vi "Read Module Name.vi"(8 "error in (no error)":errorcluster, 11 "ADAS_IO_Template_MDO in":refnum<class "ADAS_IO_Template_MDO.lvclass">) -> (0 "error out":errorcluster, 2 "Module Name":string, 3 "ADAS_IO_Template_MDO out":refnum<class "ADAS_IO_Template_MDO.lvclass">)   [LabVIEW 2020, in "ADAS_IO_Template_MDO.lvclass"]
uses:
  ADAS_IO_Template_MDO.lvclass
  ADAS_IO_Template_MDO.lvclass/ADAS_IO_Template_MDO.ctl
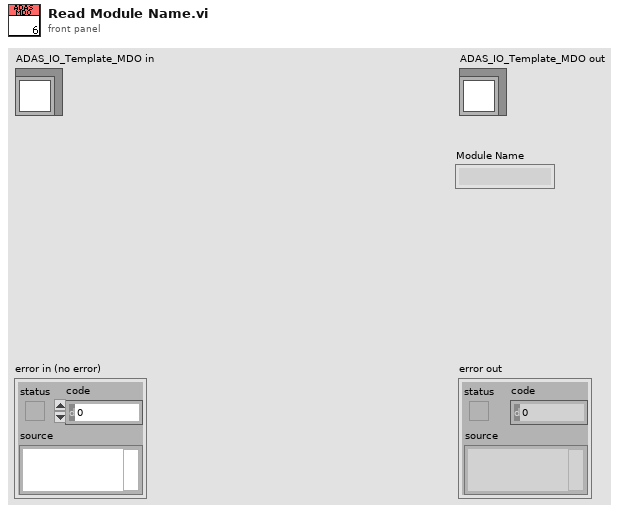
[diagram p1: front panel]
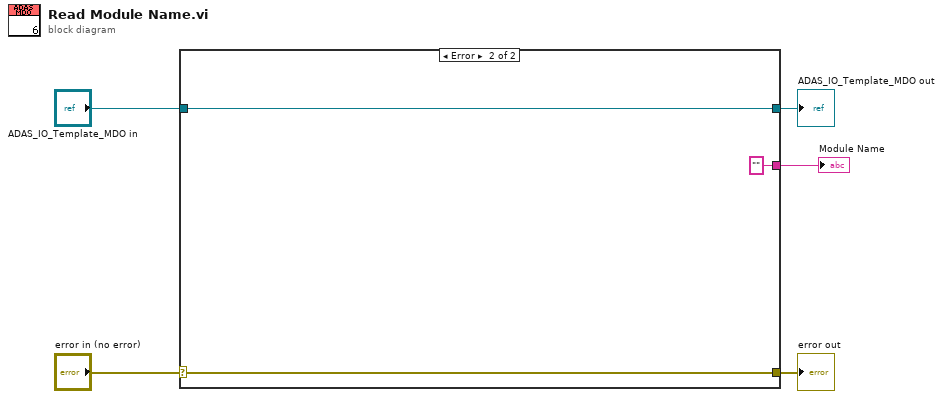
[diagram p0: block diagram]
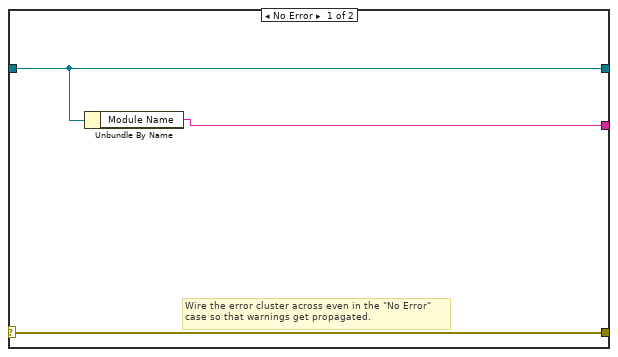
[diagram p2: hidden frame]
diagram:
  n1 = case shown="Error" "error in (no error)" {
    selector: "error in (no error)" -> [w8 w11]
    tunnel: [w8 w11] -> w4
    tunnel: [w7 w10] -> w2
    tunnel: "ADAS_IO_Template_MDO in" -> [w7 w10]
    tunnel: [w6 "" ("Module Name")] -> w1
    frame No Error {
      # "Wire the error cluster across even in the \"No Error\"\ncase so that warnings get propagated."
      n2 = Unbundle By Name(w7) -> ("Module Name"=w6:string)
    }
    frame Error {
    }
  }
  "error out" <- w4
  "ADAS_IO_Template_MDO out" <- w2
  "Module Name" <- w1
